vi "AddPathPrefix2RelPath.vi"(2 "Path":path, 3 "Path prefix":path) -> (0 "Path out":path, 1 "file or folder exists?":bool)   [LabVIEW 2016, in "Common.lvlib"]
uses:
  <userlib>/Common Components/Common/Common.lvlib
panel:
  # "if empty or not a path, the prefix is default to Application Directory"
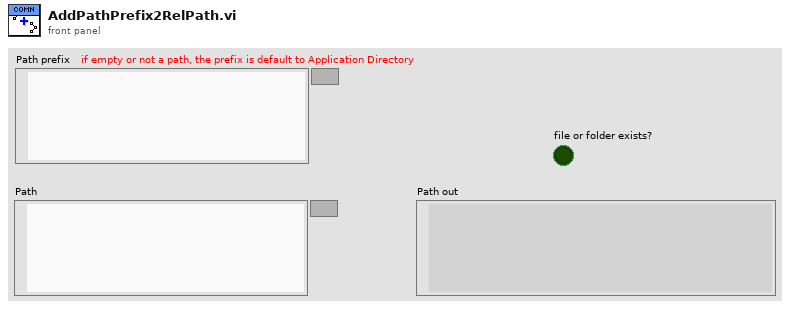
[diagram p1: front panel]
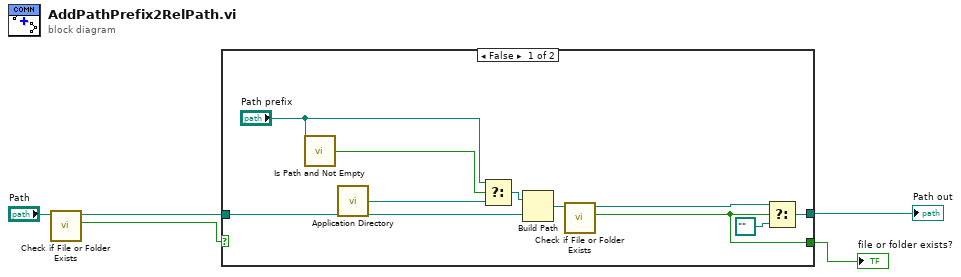
[diagram p0: block diagram]
diagram:
  n1 = call <vilib>:"Check if File or Folder Exists.vi"("path"="Path") -> ("file or folder exists?"=w3:bool, "dup path"=w1:path)  [unwired: 8 in, 1 out]
  n2 = case shown="False" w3 {
    selector: w3 -> [_ w17]
    tunnel: [w11 w17] -> w5
    tunnel: w1 -> [w14 w16]
    tunnel: [w12 w16] -> w2
    frame False {
      n3 = call <vilib>:"Is Path and Not Empty.vi"("path"="Path prefix") -> ("Is Path and Not Empty?"=w9:bool)  [unwired: 4 in]
      n4 = call <vilib>:"Application Directory.vi"() -> ("Application Directory"=w7:path)
      n5 = Select(t="Path prefix", s=w9, f=w7) -> (s? t:f=w6:path)
      n6 = Build Path(base path=w6, name or relative path=w14) -> (appended path=w15:path)
      n7 = call <vilib>:"Check if File or Folder Exists.vi"("path"=w15) -> ("file or folder exists?"=w11:bool, "dup path"=w13:path)  [unwired: 8 in, 1 out]
      n8 = Select(t=w13, s=w11, f=path "") -> (s? t:f=w12:path)
    }
    frame True {
    }
  }
  "file or folder exists?" <- w5
  "Path out" <- w2
